vi "FolderParser.vi"(1 "Folder":path) -> (0 "TreeItems[]":T1(array[cluster]))   [LabVIEW 2021, in "Tree.lvlib" / "Tree.lvclass"]
uses:
  Tree.lvclass
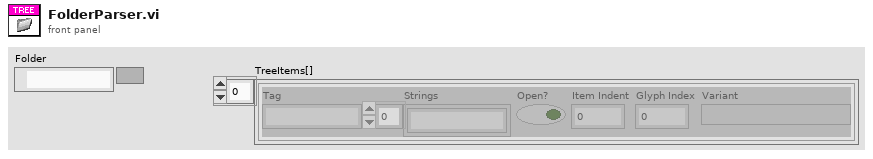
[diagram p1: front panel]
types:
  T1 = cluster{"Tag":string, "Strings":string[], "Open?":bool, "Item Indent":i32, "Glyph Index":i32, "Variant":variant}[]
  T2 = cluster{"Left Cell String":string, "Child Text":string[], "Child Tag":string, "Item Indent":i32, "Child Only?":bool, "Glyph Index":i32}[]
  T3 = cluster{"Tag":string, "Strings":string[], "Open?":bool, "Item Indent":i32, "Glyph Index":i32, "Variant":variant}
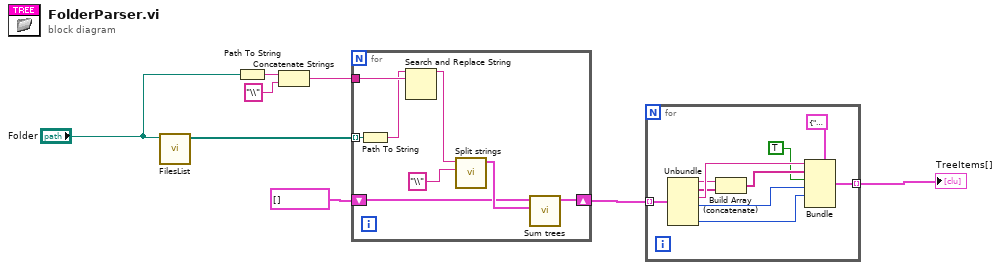
[diagram p0: block diagram]
diagram:
  n1 = call "FilesList.vi"("start path"="Folder") -> ("Array"=w4:path[])  [unwired: 9 in, 1 out]
  n2 = Path To String(path="Folder") -> (string=w6:string)
  n3 = Concatenate Strings(w6, "\\" ("regular expression")) -> (w7:string)
  n4 = for {
    shift-right: [w14] -> w2
    shift-left: T2 [] ("Tree out") -> [w13]
    tunnel: w4 -> [w12] mode=indexing
    tunnel: w7 -> [w11]
    n5 = Path To String(path=w12) -> (string=w10:string)
    n6 = Search and Replace String(input string=w10, search string=w11) -> (result string=w9:string)  [unwired: 6 in, 3 out]
    n7 = call "Split strings.vi"("regular expression"="\\", "qualified name"=w9) -> ("Arr"=w15:T2)  [unwired: 9 in]
    n8 = call "Sum trees.vi"("Add_to_tree"=w15, "Tree"=w13) -> ("Tree out"=w14:T2)  [unwired: 9 in]
  }
  n9 = for {
    tunnel: w2 -> [w26] mode=indexing
    tunnel: [w17] -> w1 mode=indexing
    n10 = Unbundle(w26) -> ("Left Cell String"=w23:string, "Child Text"=w22:string[], "Child Tag"=w24:string, "Item Indent"=w19:i32, "Glyph Index"=w20:i32)  [unwired: 1 out]
    n11 = Build Array (concatenate)(w23, w22) -> (w21:string[])
    n12 = Bundle(cluster=T3 {"Tag"="", "Strings"=[], "Open?"=FALSE, "Item Indent"=0, "Glyph Index"=0, "Variant"=variant} ("TreeItems[]"), "Tag"=w24, "Strings"=w21, "Open?"=TRUE, "Item Indent"=w19, "Glyph Index"=w20) -> (w17:T3)  [unwired: 1 in]
  }
  "TreeItems[]" <- w1
